vi "PicoScope6000WrapSettings.vi"(7 "Device Info":T1, 8 "error in (no error)":errorcluster, 9 "enabledChannels":i16[](array[numeric]), 11 "Handle In":i16) -> (0 "error out":errorcluster, 3 "Handle Out":i16)   [LabVIEW 2009]
uses:
  ps6000Wrap.dll
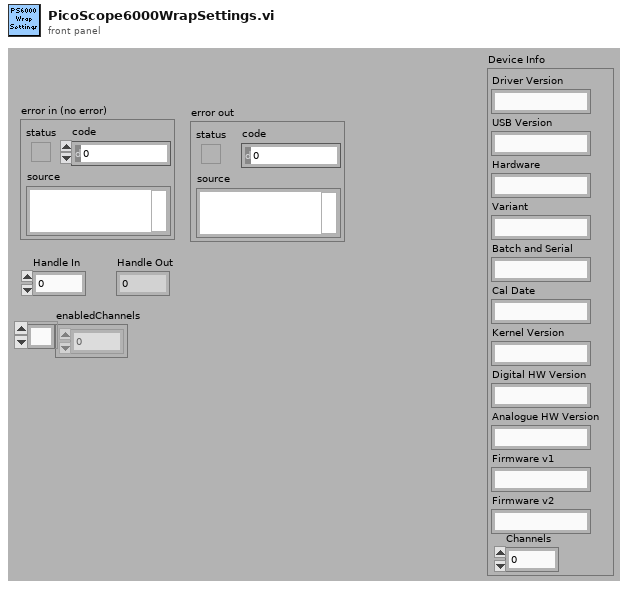
[diagram p1: front panel]
types:
  T1 = cluster{"Driver Version":string, "USB Version":string, "Hardware":string, "Variant":string, "Batch and Serial":string, "Cal Date":string, "Kernel Version":string, "Digital HW Version":string, "Analogue HW Version":string, "Firmware v1":string, "Firmware v2":string, "Channels":i16}
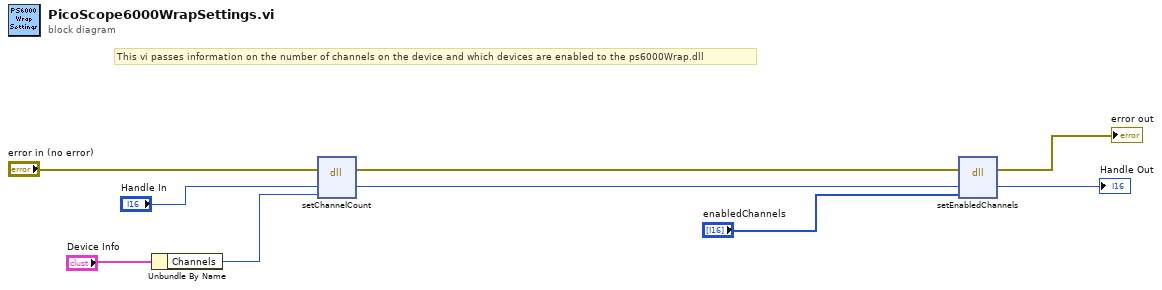
[diagram p0: block diagram]
diagram:
  # "This vi passes information on the number of channels on the device and which devices are enabled to the ps6000Wrap.dll"
  n1 = Unbundle By Name("Device Info") -> ("Channels"=w1:i16)
  n2 = dll-call lib="ps6000Wrap.dll" fn="setChannelCount"(error in="error in (no error)", "handle"="Handle In", "channelCount"=w1) -> (error out=w7:errorcluster, "handle"=w5:i16)  [unwired: 4 in, 1 out]
  n3 = dll-call lib="ps6000Wrap.dll" fn="setEnabledChannels"(error in=w7, "handle"=w5, "enabledChannels"="enabledChannels") -> (error out=→"error out":errorcluster, "handle"=→"Handle Out":i16)  [unwired: 4 in, 1 out]
